vi "Data Logging using TDMS with mult groups.vi"() -> ()   [LabVIEW 2011]
panel:
  out "Rel Time":dbl
  in  "Event":bool
  in  "stop":bool
  out "output row":dbl[](array[numeric])
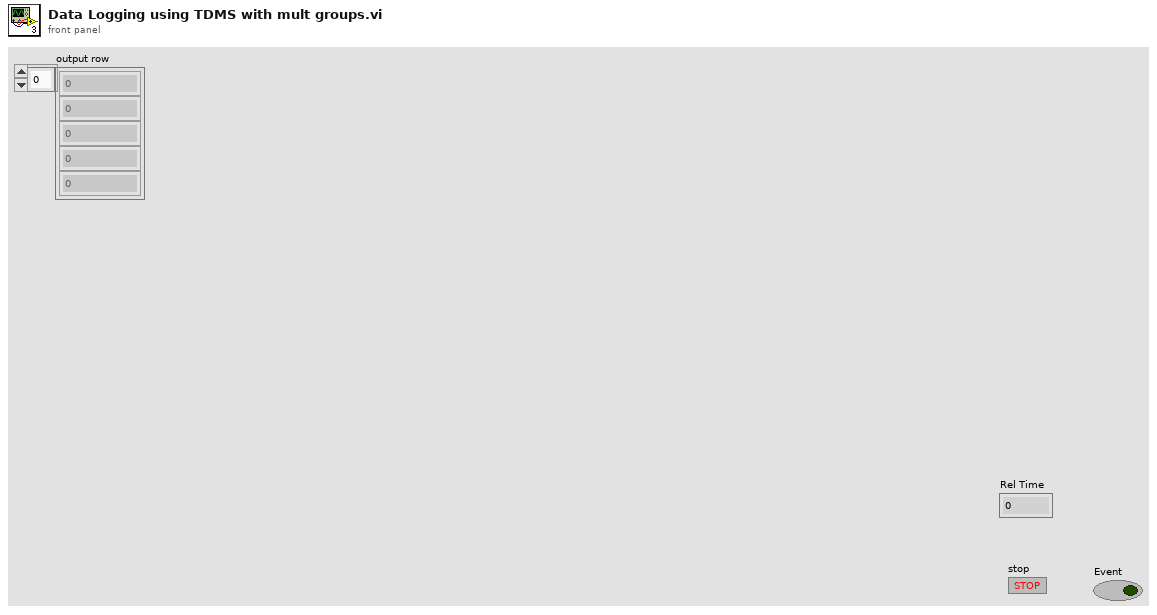
[diagram p1: front panel]
types:
  T1 = enum16{"open", "open or create", "create or replace", "create", "open (read-only)"}
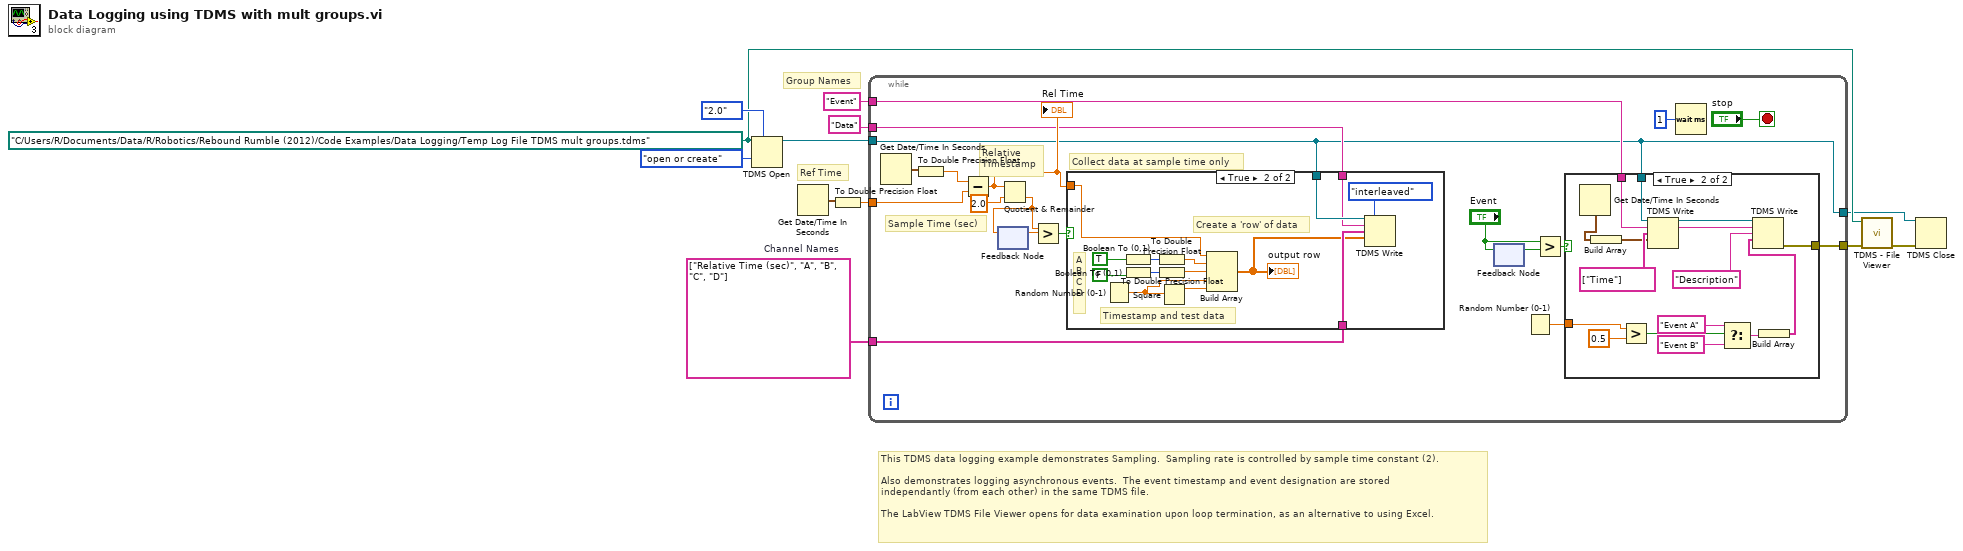
[diagram p0: block diagram]
diagram:
  w8 = string[] ["Relative Time (sec)", "A", "B", "C", "D"]  # Channel Names
  w5 = path "C:/Users/R/Documents/Data/R/Robotics/Rebound Rumble (2012)/Code Examples/Data Logging/Temp Log File TDMS mult groups.tdms" ("file path")
  # "This TDMS data logging example demonstrates Sampling.  Sampling rate is controlled by sample time constant (2).\n\nAlso demonstrates logging asynchronous events.  The event timestamp and event designation are stored\nindependantly (from each other) in the same TDMS file.\n\nThe LabView TDMS File Viewer opens for data examination upon loop termination, as an alternative to using Excel."
  # "Group Names"
  # "Ref Time"
  n1 = TDMS Open(7:enum16{"1.0", "2.0"}."2.0" ("file format version (2.0)"), 10:T1."open or create" ("operation (0:open)"), 11:w5) -> (3:w4:refnum<k34>)  [unwired: 3 in, 1 out]
  n2 = Get Date/Time In Seconds() -> (seconds since 1Jan1904=w12:timestamp)
  n3 = To Double Precision Float(number=w12) -> (double precision float=w11:dbl)
  n4 = while {
    tunnel: w11 -> [w26]
    tunnel: w4 -> [w13]
    tunnel: w8 -> [w30]
    tunnel: "Data" ("group name in (Untitled)") -> [w15]
    tunnel: [w16] -> w6
    tunnel: "Event" ("group name in (Untitled)") -> [w14]
    tunnel: [w13] -> w1
    stop <- "stop" stop-if-true
    # "Collect data at sample time only"
    # "Sample Time (sec)"
    # "Relative\nTimestamp"
    n5 = Get Date/Time In Seconds() -> (seconds since 1Jan1904=w28:timestamp)
    n6 = To Double Precision Float(number=w28) -> (double precision float=w27:dbl)
    n7 = Subtract(x=w27, y=w26) -> (x-y=w20:dbl)
    "Rel Time" <- w20
    n8 = feedback #1() -> (w23:dbl)  [unwired: 1 in]
    n9 = Quotient & Remainder(x=w20, y=2.0) -> (floor(x/y)=w22:dbl)  [unwired: 1 out]
    n10 = feedback-in #1(w22) -> ()
    n11 = Greater?(x=w22, y=w23) -> (0:w24:bool)
    n12 = case shown="True" w24 {
      tunnel: w13 -> [_ w57]
      tunnel: w15 -> [_ w56]
      tunnel: w30 -> [_ w54]
      tunnel: w20 -> [_ w51]
      frame False {
      }
      frame True {
        # "A\nB\nC\nD"
        # "Create a 'row' of data"
        # "Timestamp and test data"
        n13 = Random Number (0-1)() -> (number: 0 to 1=w49:dbl)
        n14 = Boolean To (0,1)(Boolean=TRUE) -> (0, 1=w60:i16)
        n15 = Boolean To (0,1)(Boolean=FALSE) -> (0, 1=w61:i16)
        n16 = To Double Precision Float(number=w60) -> (double precision float=w53:dbl)
        n17 = To Double Precision Float(number=w61) -> (double precision float=w52:dbl)
        n18 = Square(x=w49) -> (x^2=w48:dbl)
        n19 = Build Array(w51, w53, w52, w49, w48) -> (w50:dbl[])
        "output row" <- w50
        n20 = TDMS Write(0:w57, 1:enum16{"decimated", "interleaved"}."interleaved" ("data layout (0:decimated)"), 5:w56, 7:w54, 9:w50) -> ()  [unwired: 1 in, 4 out]
      }
    }
    n21 = feedback-in #2("Event") -> ()
    n22 = feedback #2() -> (w18:bool)  [unwired: 1 in]
    n23 = Random Number (0-1)() -> (number: 0 to 1=w21:dbl)
    n24 = Greater?(x="Event", y=w18) -> (0:w19:bool)
    n25 = case shown="True" w19 {
      tunnel: w13 -> [_ w47]
      tunnel: w21 -> [_ w40]
      tunnel: [_ w33] -> w16
      tunnel: w14 -> [_ w32]
      frame False {
      }
      frame True {
        n26 = Get Date/Time In Seconds() -> (seconds since 1Jan1904=w42:timestamp)
        n27 = Build Array(w42) -> (w43:timestamp[])
        n28 = Greater?(x=w40, y=0.5) -> (0:w39:bool)
        n29 = TDMS Write(0:w47, 5:w32, 7:string[] ["Time"] ("channel name(s) in (Untitled)"), 9:w43) -> (4:w46:refnum<k34>, 6:w45:string)  [unwired: 2 in, 2 out]
        n30 = Select(t="Event A", s=w39, f="Event B") -> (s? t:f=w34:string)
        n31 = Build Array(w34) -> (w36:string[])
        n32 = TDMS Write(0:w46, 5:w45, 7:"Description" ("channel name(s) in (Untitled)"), 9:w36) -> (15:w33:errorcluster)  [unwired: 2 in, 3 out]
      }
    }
    n33 = Wait (ms)(milliseconds to wait=u32 1) -> ()  [unwired: 1 out]
  }
  n34 = call <vilib>:"TDMS - File Viewer.vi"("error in (no error)"=w6, "file path"=w5) -> ("error out"=w2:errorcluster)  [unwired: 4 in, 1 out]
  n35 = TDMS Close(8:w2, 11:w1) -> ()  [unwired: 2 out]
